vi "Arieh Temp.vi"() -> ()   [LabVIEW 2015]
uses:
  <vilib>/FPGAPlugInAG/cRIO-9030/niLvFpga_Open_cRIO-9030.vi
  <vilib>/rvi/interface/common/dynamic/niFpgaDynamicAddResources.vi
  <vilib>/FPGAPlugInAG/Dynamic/niLvFpga_Run_Dynamic.vi
  <vilib>/Utility/error.llb/Error Cluster From Error Code.vi
  <vilib>/rvi/errors/niLvFpgaAdjustHostInterfaceError.vi
  <vilib>/rvi/interface/nirviOpenFPGA/nirviOpenFPGA.xnode
  FPGA Bitfiles/BELKINEAGLEGUI_FPGATarget_EagleFPGAScanner_AddXN+PC+cM.lvbitx
  Eagle_FPGA Scanner Control.vi
  <vilib>/rvi/interface/nirviMethod/nirviMethod.xnode
  <vilib>/rvi/interface/nirviReadWriteControl/nirviReadWriteControl.xnode
  NiFpgaLv.dll
  <vilib>/rvi/interface/Simulation/niFpgaSimulationCallBeginRW.vi
  IP Dev Area/IP results.ctl
panel:
  out "Y min value":dbl
  out "Y max value":dbl
  out "X min value":dbl
  out "X max value":dbl
  out "XY Graph":cluster{"PX":dbl[], "PY":dbl[]}(graph)
  in  "Y Multi":dbl=0.006666 format="%#_13g"
  in  "Y Offs":dbl=-2.0 format="%#_13g"
  out "Y":dbl[](array[numeric])
  out "X":dbl[](array[numeric])
  in  "X Offs":dbl=-2.0 format="%#_13g"
  in  "X Multi":dbl=0.005 format="%#_13g"
  out "PY":fxp<+,10,10>[](array[numeric])
  out "PX":fxp<+,10,10>[](array[numeric])
  in  "Radius B":fxp<+/-,10,10>=180.0
  in  "Radius A":fxp<+/-,10,10>=180.0
  in  "Center":T1={"CX"=400.0, "CY"=300.0}
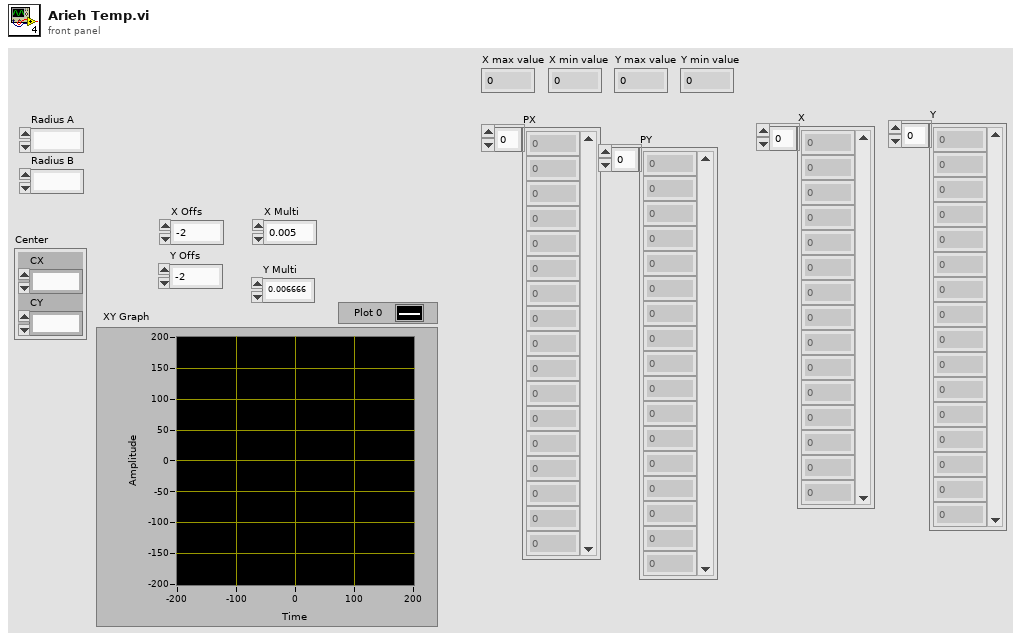
[diagram p1: front panel]
types:
  T1 = cluster{"CX":fxp<+/-,10,10>, "CY":fxp<+/-,10,10>}
  T2 = cluster{"PxMin":fxp<+,10,10>, "PxMax":fxp<+,10,10>, "PyMin":fxp<+,10,10>, "PyMax":fxp<+,10,10>}
  T3 = cluster{"X MULT":fxp<+/-,20,5>, "Y MULT":fxp<+/-,20,5>, "X OFFS":fxp<+/-,20,5>, "Y OFFS":fxp<+/-,20,5>}
  T4 = typedef "IP results.ctl" = cluster{"X":u16, "Y":u16, "A":dbl, "B":dbl, "Grade":u16, "Frame#":u16}
  T5 = cluster{"PX":fxp<+,10,10>[], "PY":fxp<+,10,10>[]}
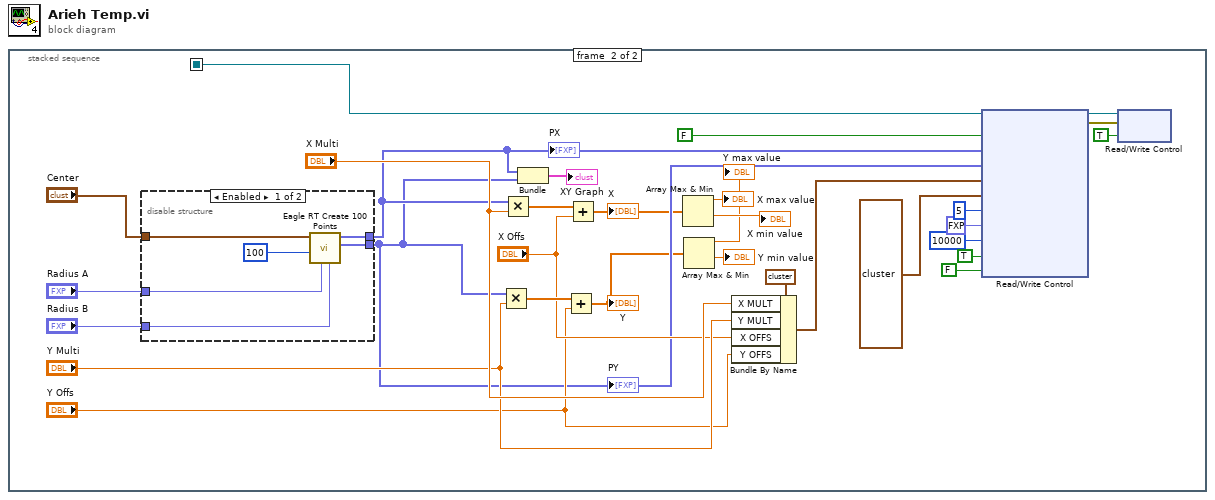
[diagram p0: block diagram]
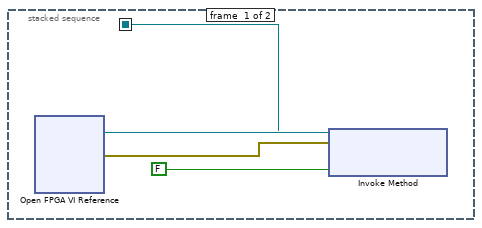
[diagram p2: hidden frame]
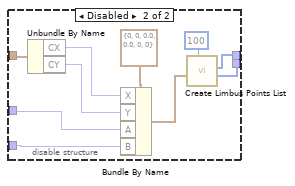
[diagram p3: hidden frame]
diagram:
  n1 = stacked-sequence {
    seq-local: [w1 _] -> [_ w30]
    frame #0 {
      n2 = xnode "Open FPGA VI Reference"() -> ("FPGA VI Reference Out"=w4:refnum<k20>, "error out"=w3:errorcluster)  [unwired: 2 in]
      n3 = xnode "Invoke Method"("FPGA VI Reference In"=w4, "error in"=w3, "Wait Until Done (F)"=FALSE) -> ("FPGA VI Reference Out"=w1:refnum<k20>)  [unwired: 1 out]
    }
    frame #1 {
      n4 = disable-structure shown="Enabled" {
        disable-tunnel: "Center" -> [w41 w46]
        disable-tunnel: "Radius A" -> [w39 w43]
        disable-tunnel: "Radius B" -> [w38 w42]
        disable-tunnel: [w37 w48] -> w15
        disable-tunnel: [w36 w47] -> w14
        frame Enabled {
          n5 = call "Eagle RT Create 100 Points.vi"("Radius B"=w38, "Radius A"=w39, "NumOfPoints"=100, "Center"=w41) -> ("PY"=w36:fxp<+,10,10>[], "PX"=w37:fxp<+,10,10>[])  [unwired: 6 in]
        }
        frame Disabled {
          n6 = Unbundle By Name(w46) -> ("CX"=w45:fxp<+/-,10,10>, "CY"=w44:fxp<+/-,10,10>)
          n7 = Bundle By Name(cluster=T4 {"X"=0, "Y"=0, "A"=0.0, "B"=0.0, "Grade"=0, "Frame#"=0} ("IP Results"), "X"=w45, "Y"=w44, "A"=w43, "B"=w42) -> (w49:T4)
          n8 = call "Create Limbus Points List.vi"("NoOfPoints"=u16 100, "IP Results"=w49) -> ("Y Points"=w47:i16[], "X Points"=w48:i16[])  [unwired: 8 in]
        }
      }
      "PX" <- w15
      "PY" <- w14
      n9 = Multiply(x=w14, y="Y Multi") -> (x*y=w31:dbl[])
      n10 = Multiply(x=w15, y="X Multi") -> (x*y=w32:dbl[])
      n11 = Bundle("PX"=w15, "PY"=w14) -> (→"XY Graph":T5)  [unwired: 1 in]
      n12 = Add(x=w31, y="Y Offs") -> (x+y=w9:dbl[])
      "Y" <- w9
      n13 = Add(x=w32, y="X Offs") -> (x+y=w12:dbl[])
      "X" <- w12
      n14 = Array Max & Min(array=w12) -> (max value=→"X max value":dbl, min value=→"X min value":dbl)  [unwired: 2 out]
      n15 = Array Max & Min(array=w9) -> (max value=→"Y max value":dbl, min value=→"Y min value":dbl)  [unwired: 2 out]
      n16 = Bundle By Name(cluster=T3 {"X MULT"=0.0, "Y MULT"=0.0, "X OFFS"=0.0, "Y OFFS"=0.0} ("Calib Values"), "X MULT"="X Multi", "Y MULT"="Y Multi", "X OFFS"="X Offs", "Y OFFS"="Y Offs") -> (w27:T3)
      n17 = xnode "Read/Write Control"("FPGA VI Reference In"=w30, "Manual"=FALSE, "X Array"=w15, "Y Array"=w14, "Calib Values"=w27, "NoGO Zone"=T2 {"PxMin"=400.0, "PxMax"=400.0, "PyMin"=300.0, "PyMax"=300.0}, "NumOfRetries"=u16 5, "Aim Ctrl"=fxp<+,16,3> 0.0, "ScanRate"=u32 10000, "Illumination_Ena"=TRUE, "One Shot"=FALSE) -> ("FPGA VI Reference Out"=w20:refnum<k20>, "error out"=w19:errorcluster)  [unwired: 1 in]
      n18 = xnode "Read/Write Control"("FPGA VI Reference In"=w20, "error in"=w19, "Enable"=TRUE ("Reset")) -> ()  [unwired: 2 out]
    }
  }
